vi "Search_RemoveFrom_Database.vi"(11 "Database In":T1[](array[typedef])) -> (3 "Database Out":T1[](array[typedef]))   [LabVIEW 2022 SP3]
uses:
  Database_element.ctl
  91c73ffb-74ba-43a8-a4f4-807e3001293a.vi
  443cf8cf-0bae-4e46-884c-996c58ab8b2d.vi
  ae07310f-4d48-47c8-8365-1d528dd077b0.vi
  b768ac9d-5475-4889-9179-c41377d87a59.vi
  228d6626-65a0-4d62-936b-05c5f66c30d4.vi
  cd490f5d-371c-4503-aa22-744dd188d3dd.vi
  1b63c330-6ec9-49cf-b997-f1ce1cff0b75.vi
  f64d8d88-4023-43dd-bf67-7aa74b69d8d9.vi
  e7812817-1b2b-4492-8f61-9f9b99c972cb.vi
  <vilib>/Array/Sort 2D Array - Pop Stack.vi
  <vilib>/Array/Sort 2D Array - Push Stack.vi
panel:
  in  "Array 2":bool[](array[boolean])=[FALSE, FALSE, FALSE, FALSE, FALSE, FALSE, FALSE, FALSE, FALSE, FALSE, FALSE]
  out "Array":string[](array[string])
  in  "Close":bool
  in  "Sort By:":T2(ring)
  in  "Search By:":T2(ring)
  in  "Search":string
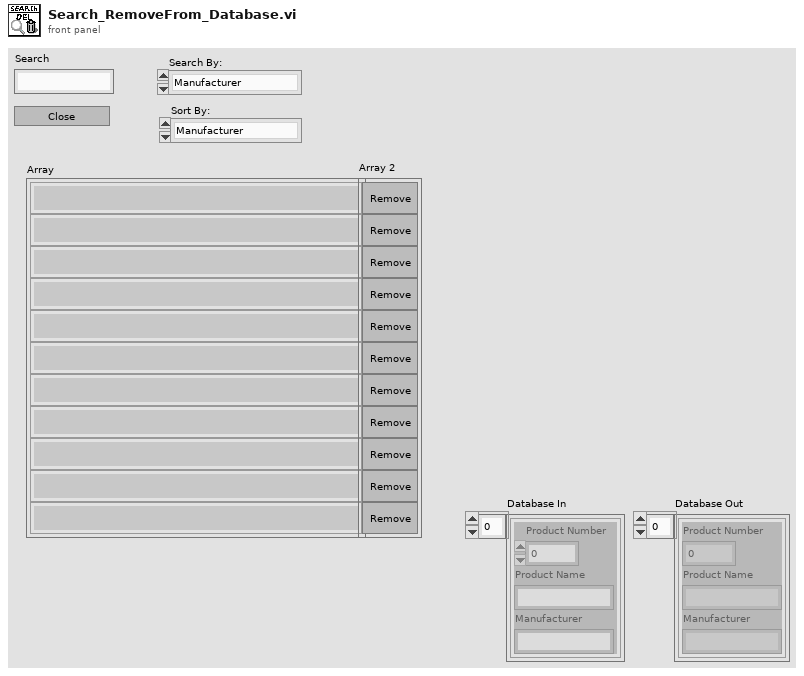
[diagram p1: front panel]
types:
  T1 = typedef "Database_element.ctl" = cluster{"Product Number":i32, "Product Name":string, "Manufacturer":string}
  T2 = enum16{"Manufacturer", "Product Name", "Product Number"}
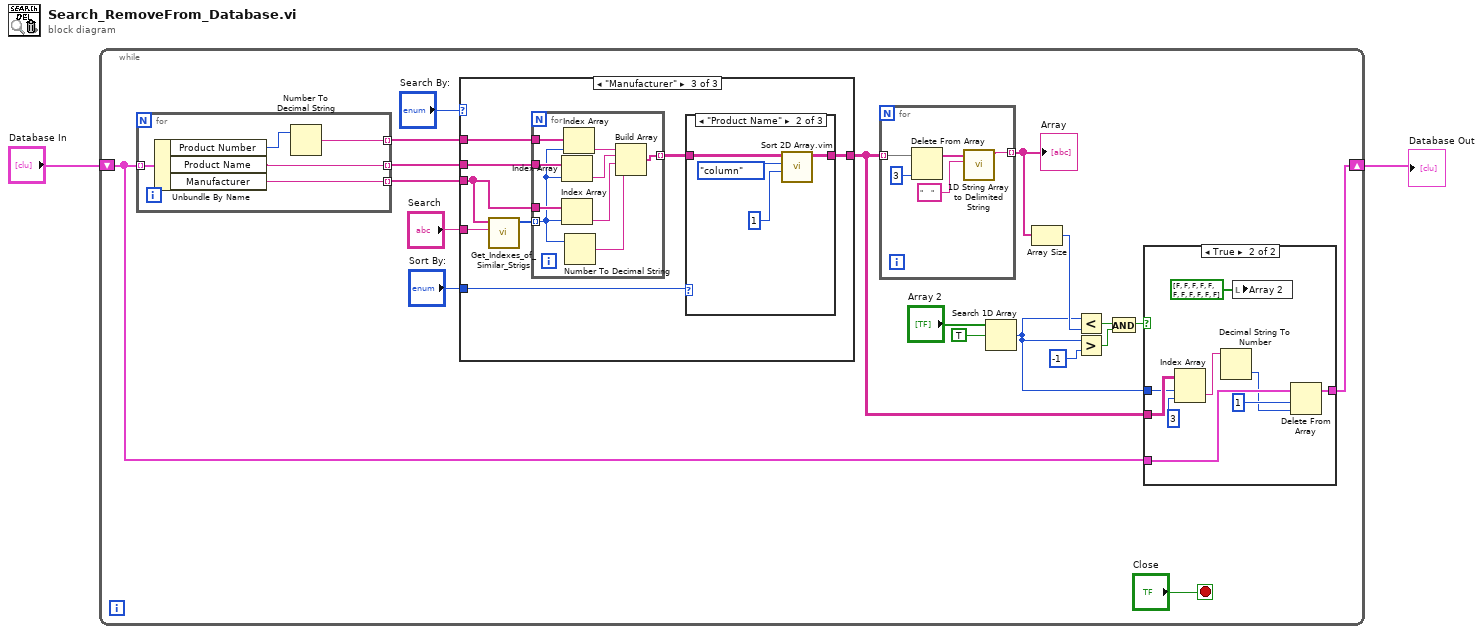
[diagram p0: block diagram]
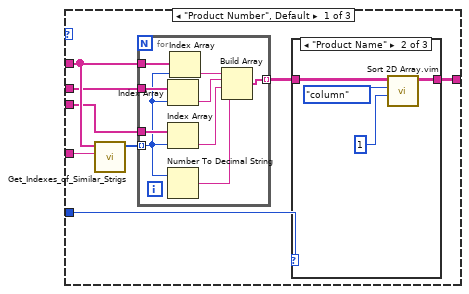
[diagram p3: hidden frame]
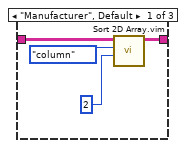
[diagram p4: hidden frame]
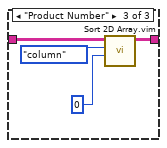
[diagram p5: hidden frame]
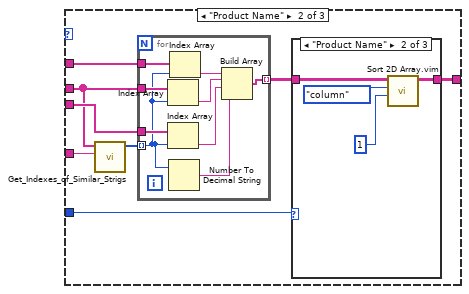
[diagram p6: hidden frame]
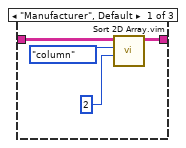
[diagram p7: hidden frame]
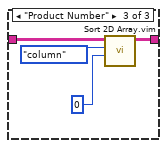
[diagram p8: hidden frame]
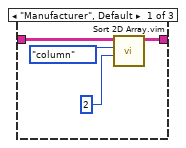
[diagram p9: hidden frame]
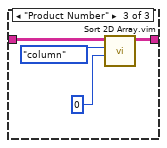
[diagram p10: hidden frame]
diagram:
  n1 = while {
    shift-right: [w3] -> w1
    shift-left: "Database In" -> [w6]
    stop <- "Close" stop-if-true
    n2 = for {
      tunnel: w6 -> [w41] mode=indexing
      tunnel: [w40] -> w17 mode=indexing
      tunnel: [w39] -> w16 mode=indexing
      tunnel: [w37] -> w15 mode=indexing
      n3 = Unbundle By Name(w41) -> ("Product Number"=w38:i32, "Product Name"=w40:string, "Manufacturer"=w39:string)
      n4 = Number To Decimal String(number=w38) -> (decimal integer string=w37:string)  [unwired: 1 in]
    }
    n5 = case shown="\"Manufacturer\"" "Search By:" {
      tunnel: w15 -> [w47 w76 w105]
      tunnel: "Search" -> [w49 w78 w107]
      tunnel: w17 -> [w46 w71 w101]
      tunnel: w16 -> [w45 w75 w100]
      tunnel: "Sort By:" -> [w44 w74 w104]
      tunnel: [w42 w72 w102] -> w5
      frame "Product Number", Default {
        n6 = call "Get_Indexes_of_Similar_Strigs.vi"("Search"=w49, "Input 1D array"=w47) -> ("Indexes"=w48:i32[])  [unwired: 9 in]
        n7 = for {
          tunnel: w48 -> [w63] mode=indexing
          tunnel: w47 -> [w70]
          tunnel: w46 -> [w69]
          tunnel: w45 -> [w68]
          tunnel: [w64] -> w43 mode=indexing
          n8 = Index Array(array=w69, index=w63) -> (element=w66:string)
          n9 = Index Array(array=w68, index=w63) -> (element=w65:string)
          n10 = Number To Decimal String(number=w63) -> (decimal integer string=w62:string)  [unwired: 1 in]
          n11 = Index Array(array=w70, index=w63) -> (element=w67:string)
          n12 = Build Array(w67, w66, w65, w62) -> (w64:string[])
        }
        n13 = case shown="\"Product Name\"" w44 {
          tunnel: w43 -> [w53 w57 w61]
          tunnel: [w50 w54 w58] -> w42
          frame "Manufacturer", Default {
            n14 = call "Sort 2D Array.vim"("index"=2, "dimension to index (column)"=enum16{"column", "row"}."column", "2D array"=w53) -> ("sorted 2D array"=w50:string[][])  [unwired: 7 in, 1 out]
          }
          frame "Product Name" {
            n15 = call "Sort 2D Array.vim"("index"=1, "dimension to index (column)"=enum16{"column", "row"}."column", "2D array"=w57) -> ("sorted 2D array"=w54:string[][])  [unwired: 7 in, 1 out]
          }
          frame "Product Number" {
            n16 = call "Sort 2D Array.vim"("index"=0, "dimension to index (column)"=enum16{"column", "row"}."column", "2D array"=w61) -> ("sorted 2D array"=w58:string[][])  [unwired: 7 in, 1 out]
          }
        }
      }
      frame "Product Name" {
        n17 = call "Get_Indexes_of_Similar_Strigs.vi"("Search"=w78, "Input 1D array"=w71) -> ("Indexes"=w77:i32[])  [unwired: 9 in]
        n18 = for {
          tunnel: w77 -> [w92] mode=indexing
          tunnel: w76 -> [w99]
          tunnel: w71 -> [w98]
          tunnel: w75 -> [w97]
          tunnel: [w93] -> w73 mode=indexing
          n19 = Index Array(array=w98, index=w92) -> (element=w95:string)
          n20 = Index Array(array=w97, index=w92) -> (element=w94:string)
          n21 = Number To Decimal String(number=w92) -> (decimal integer string=w91:string)  [unwired: 1 in]
          n22 = Index Array(array=w99, index=w92) -> (element=w96:string)
          n23 = Build Array(w96, w95, w94, w91) -> (w93:string[])
        }
        n24 = case shown="\"Product Name\"" w74 {
          tunnel: w73 -> [w82 w86 w90]
          tunnel: [w79 w83 w87] -> w72
          frame "Manufacturer", Default {
            n25 = call "Sort 2D Array.vim"("index"=2, "dimension to index (column)"=enum16{"column", "row"}."column", "2D array"=w82) -> ("sorted 2D array"=w79:string[][])  [unwired: 7 in, 1 out]
          }
          frame "Product Name" {
            n26 = call "Sort 2D Array.vim"("index"=1, "dimension to index (column)"=enum16{"column", "row"}."column", "2D array"=w86) -> ("sorted 2D array"=w83:string[][])  [unwired: 7 in, 1 out]
          }
          frame "Product Number" {
            n27 = call "Sort 2D Array.vim"("index"=0, "dimension to index (column)"=enum16{"column", "row"}."column", "2D array"=w90) -> ("sorted 2D array"=w87:string[][])  [unwired: 7 in, 1 out]
          }
        }
      }
      frame "Manufacturer" {
        n28 = call "Get_Indexes_of_Similar_Strigs.vi"("Search"=w107, "Input 1D array"=w100) -> ("Indexes"=w106:i32[])  [unwired: 9 in]
        n29 = for {
          tunnel: w106 -> [w121] mode=indexing
          tunnel: w105 -> [w128]
          tunnel: w101 -> [w127]
          tunnel: w100 -> [w126]
          tunnel: [w122] -> w103 mode=indexing
          n30 = Index Array(array=w127, index=w121) -> (element=w124:string)
          n31 = Index Array(array=w126, index=w121) -> (element=w123:string)
          n32 = Index Array(array=w128, index=w121) -> (element=w125:string)
          n33 = Number To Decimal String(number=w121) -> (decimal integer string=w120:string)  [unwired: 1 in]
          n34 = Build Array(w125, w124, w123, w120) -> (w122:string[])
        }
        n35 = case shown="\"Product Name\"" w104 {
          tunnel: w103 -> [w111 w115 w119]
          tunnel: [w108 w112 w116] -> w102
          frame "Manufacturer", Default {
            n36 = call "Sort 2D Array.vim"("index"=2, "dimension to index (column)"=enum16{"column", "row"}."column", "2D array"=w111) -> ("sorted 2D array"=w108:string[][])  [unwired: 7 in, 1 out]
          }
          frame "Product Name" {
            n37 = call "Sort 2D Array.vim"("index"=1, "dimension to index (column)"=enum16{"column", "row"}."column", "2D array"=w115) -> ("sorted 2D array"=w112:string[][])  [unwired: 7 in, 1 out]
          }
          frame "Product Number" {
            n38 = call "Sort 2D Array.vim"("index"=0, "dimension to index (column)"=enum16{"column", "row"}."column", "2D array"=w119) -> ("sorted 2D array"=w116:string[][])  [unwired: 7 in, 1 out]
          }
        }
      }
    }
    n39 = for {
      tunnel: w5 -> [w36] mode=indexing
      tunnel: [w32] -> w12 mode=indexing
      n40 = Delete From Array(array=w36, index=3) -> (array with subset deleted=w34:string[])  [unwired: 1 in, 1 out]
      n41 = call <vilib>:"1D String Array to Delimited String.vi"("delimiter"="    ", "string array"=w34) -> ("delimited string"=w32:string)  [unwired: 9 in]
    }
    "Array" <- w12
    n42 = Search 1D Array(1D array="Array 2", element=TRUE) -> (index of element=w4:i32)  [unwired: 1 in]
    n43 = Array Size(array=w12) -> (size(s)=w10:i32)
    n44 = Less?(x=w4, y=w10) -> (x < y?=w9:bool)
    n45 = Greater?(x=w4, y=-1) -> (0:w8:bool)
    n46 = And(x=w9, y=w8) -> (x .and. y?=w7:bool)
    n47 = case shown="True" w7 {
      tunnel: w6 -> [w22 w28]
      tunnel: w5 -> [_ w31]
      tunnel: w4 -> [_ w30]
      tunnel: [w22 w24] -> w3
      frame False {
      }
      frame True {
        n48 = Index Array(array=w31, index (row)=w30, index (col)=3 ("disabled index (col)")) -> (element=w26:string)
        n49 = Decimal String To Number(string=w26) -> (number=w25:i32)  [unwired: 2 in, 1 out]
        n50 = local write "Array 2"(bool[] [FALSE, FALSE, FALSE, FALSE, FALSE, FALSE, FALSE, FALSE, FALSE, FALSE, FALSE] ("Array 2")) -> ()
        n51 = Delete From Array(array=w28, length=1, index=w25) -> (array with subset deleted=w24:T1[])  [unwired: 1 out]
      }
    }
  }
  "Database Out" <- w1
